vi "Load_Template_Globals.vi"(1 "Channel Names":string[](array[string]), 2 "Template-read":path) -> (0 "Valid Template File?":bool)   [LabVIEW 2010]
uses:
  Controls/Global_mode.ctl
  Results_plotter_Global.vi
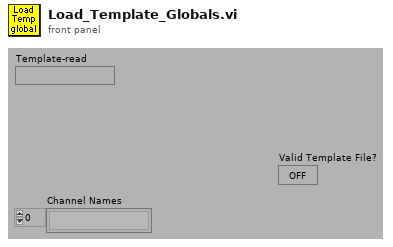
[diagram p1: front panel]
types:
  T1 = typedef "Global_mode.ctl" = enum16{"Read Global", "Load Global From File", "Write Global to File"}
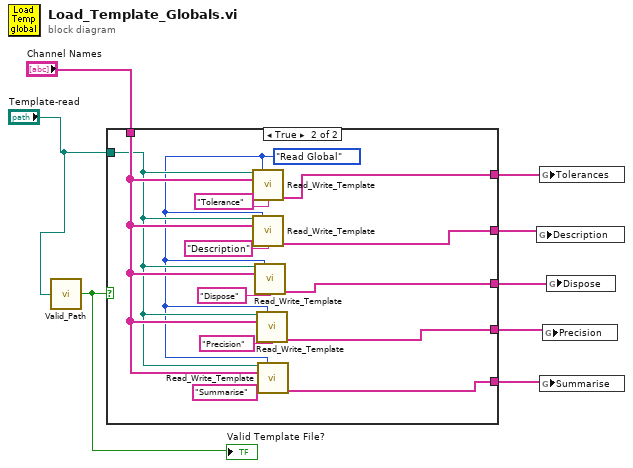
[diagram p0: block diagram]
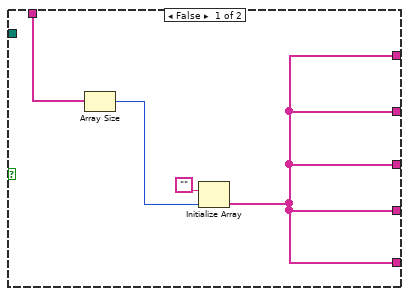
[diagram p2: hidden frame]
diagram:
  n1 = call "Valid_Path.vi"("Filename"="Template-read") -> ("Valid Path?"=w1:bool)
  "Valid Template File?" <- w1
  n2 = case shown="True" w1 {
    tunnel: "Template-read" -> [_ w15]
    tunnel: "Channel Names" -> [w11 w20]
    tunnel: [w9 w19] -> w4
    tunnel: [w9 w18] -> w5
    tunnel: [w9 w17] -> w6
    tunnel: [w9 w16] -> w7
    tunnel: [w9 w13] -> w8
    frame False {
      n3 = Array Size(array=w11) -> (size(s)=w10:i32)
      n4 = Initialize Array("", w10) -> (w9:string[])
    }
    frame True {
      w14 = Global_mode."Read Global" ("Mode")
      n5 = call "Read_Write_Template.vi"("Template File"=w15, "Mode"=w14, "Channel names In"=w20, "Data type"="Tolerance") -> ("1D Info Out"=w13:string[])  [unwired: 4 in, 7 out]
      n6 = call "Read_Write_Template.vi"("Template File"=w15, "Mode"=w14, "Channel names In"=w20, "Data type"="Description") -> ("1D Info Out"=w16:string[])  [unwired: 4 in, 7 out]
      n7 = call "Read_Write_Template.vi"("Template File"=w15, "Mode"=w14, "Channel names In"=w20, "Data type"="Dispose") -> ("1D Info Out"=w17:string[])  [unwired: 4 in, 7 out]
      n8 = call "Read_Write_Template.vi"("Template File"=w15, "Mode"=w14, "Channel names In"=w20, "Data type"="Precision") -> ("1D Info Out"=w18:string[])  [unwired: 4 in, 7 out]
      n9 = call "Read_Write_Template.vi"("Template File"=w15, "Mode"=w14, "Channel names In"=w20, "Data type"="Summarise") -> ("1D Info Out"=w19:string[])  [unwired: 4 in, 7 out]
    }
  }
  n10 = global write "Results_plotter_Global.vi" "Description"(w7) -> ()
  n11 = global write "Results_plotter_Global.vi" "Tolerances"(w8) -> ()
  n12 = global write "Results_plotter_Global.vi" "Summarise"(w4) -> ()
  n13 = global write "Results_plotter_Global.vi" "Precision"(w5) -> ()
  n14 = global write "Results_plotter_Global.vi" "Dispose"(w6) -> ()
